vi "ShowPanel.vi"(8 "error in (no error)":errorcluster, 11 "NI_DAQmx(AI) in":refnum<class "NI_DAQmx(AI).lvclass">) -> (0 "error out":errorcluster, 3 "NI_DAQmx(AI) out":refnum<class "NI_DAQmx(AI).lvclass">)   [LabVIEW 2025, in "NI_DAQmx(AI).lvclass"]
uses:
  NI_DAQmx(AI).lvclass
  D:/Hardware/DAQ/DAQ_Abstr/Task_Abstr/Task_Abstr/Task_Abstr.lvclass
  NI_DAQmx(AI).lvclass/NI_DAQmx(AI).ctl
  DAQ_Abstr/Task_Type/AI_Task/AI_Task/AI_Task.lvclass
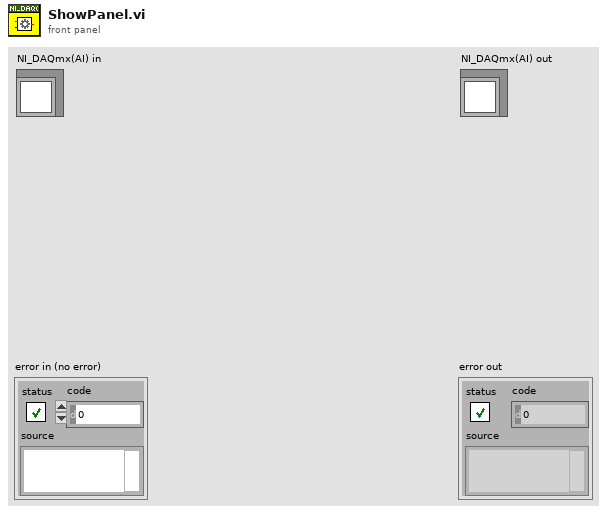
[diagram p1: front panel]
types:
  T1 = enum32{"Invalid", "Standard", "Closed", "Hidden", "Minimized", "Maximized"}
  T2 = typedef "DAQ_Module.lvlib/DAQ_Module.lvclass/DAQ_Task_Config.ctl" = cluster{"TaskType":T3, "PhysicalChannels":string, "SampleRateConfiguration":cluster{"SampleRate":dbl, "SamplesPerChannel":u32, "SamplesPerRead":i32, "SampleMode":i32, "Clock Source":string}, "ChannelConfig":string}
  T3 = typedef "DAQ_Module.lvlib/DAQ_Module.lvclass/DAQ_Task_Type.ctl" = enum16{"AI", "Linear", "Angular", "AO"}
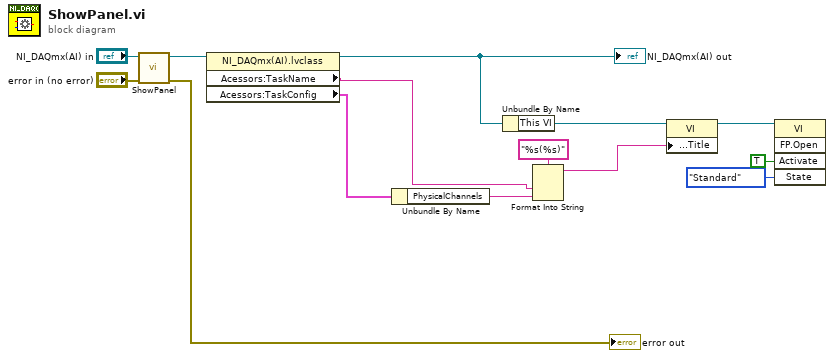
[diagram p0: block diagram]
diagram:
  n1 = call-parent "ShowPanel.vi"("error in (no error)"="error in (no error)", "Task_Abstr in"="NI_DAQmx(AI) in") -> ("error out"=→"error out":errorcluster, "Task_Abstr out"=w11:refnum<class "NI_DAQmx(AI).lvclass">)  [unwired: 8 in]
  n2 = property class="NI_DAQmx(AI).lvclass"(reference=w11) -> (reference out=w10:refnum<class "NI_DAQmx(AI).lvclass">, "Acessors:TaskName"=w2:string, "Acessors:TaskConfig"=w5:T2)  [unwired: 1 in, 1 out]
  "NI_DAQmx(AI) out" <- w10
  n3 = Unbundle By Name(w5) -> ("PhysicalChannels"=w3:string)
  n4 = Unbundle By Name(w10) -> ("This VI"=w9:refnum<vi>)
  n5 = Format Into String(format string="%s(%s)", w2, w3) -> (resulting string=w1:string)  [unwired: 2 in, 1 out]
  n6 = property class="VI"(reference=w9, "Front Panel.Title"=w1) -> (reference out=w8:refnum<vi>)  [unwired: 1 in, 1 out]
  n7 = invoke class="VI" method="FP.Open"(reference=w8, "Activate"=TRUE ("Activate?"), "State"=T1."Standard") -> ()  [unwired: 2 in, 5 out]
